vi "Get_Wavelength.vi"(8 "error in (no error)":errorcluster, 11 "Thorlabs_PM100D in":refnum<class "Thorlabs_PM100D.lvclass">) -> (0 "error out":errorcluster, 2 "Wavelength (m)":dbl, 3 "Thorlabs_PM100D out":refnum<class "Thorlabs_PM100D.lvclass">)   [LabVIEW 2020, in "Thorlabs_PM100D.lvclass"]
uses:
  <instrlib>/Classes/Powermeter/Thorlabs_PM100D/Thorlabs_PM100D.lvclass
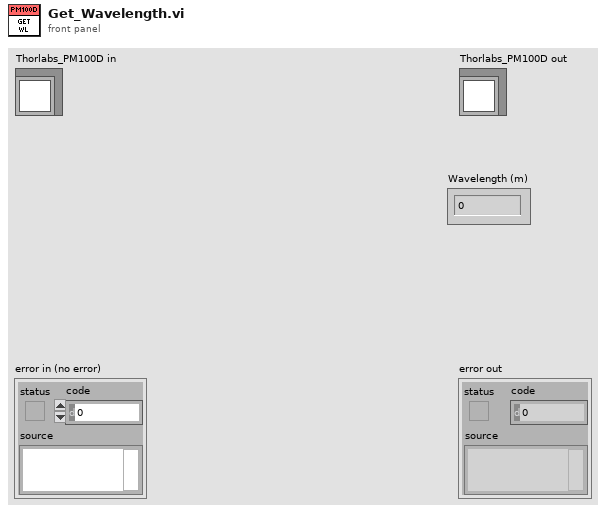
[diagram p1: front panel]
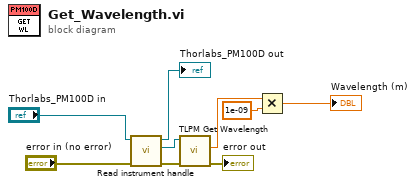
[diagram p0: block diagram]
diagram:
  n1 = call-dynamic "Read instrument handle.vi"("error in (no error)"="error in (no error)", "Thorlabs_PM100D in"="Thorlabs_PM100D in") -> ("error out"=w5:errorcluster, "instrument handle"=w6:refnum<visa-resource-name>, "Thorlabs_PM100D out"=→"Thorlabs_PM100D out":refnum<class "Thorlabs_PM100D.lvclass">)  [unwired: 7 in]
  n2 = call <instrlib>:"TLPM Get Wavelength.vi"("error in (no error)"=w5, "instrument handle"=w6) -> ("error out"=→"error out":errorcluster, "Wavelength"=w4:dbl)  [unwired: 7 in, 1 out]
  n3 = Multiply(x=w4, y=1e-09) -> (x*y=→"Wavelength (m)":dbl)
